vi "GUI Module.vi"(8 "Error In":errorcluster, 10 "GUI Types":T2=enum."Vibratome GUI", 11 "GUI Actions":T1) -> (0 "Error Out":errorcluster)   [LabVIEW 2014]
uses:
  Controls/GUI Types.ctl
  Controls/GUI Module Actions.ctl
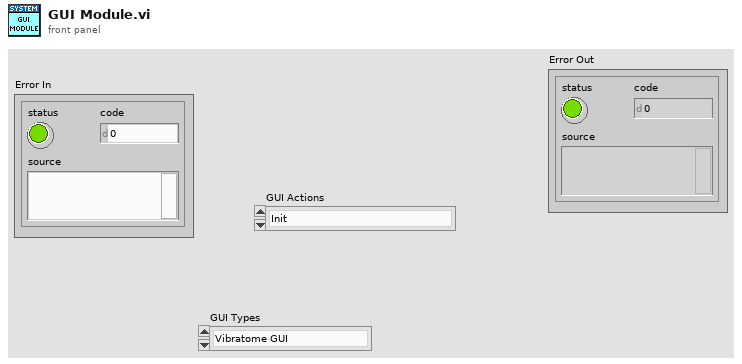
[diagram p1: front panel]
types:
  T1 = typedef "GUI Module Actions.ctl" = enum16{"Init", "Open Front Panel", "Hide All Front Panels", "Close Front Panel", "Uninit"}
  T2 = typedef "GUI Types.ctl" = enum16{"Mosaic GUI", "Vibratome GUI"}
  T3 = enum32{"Invalid", "Standard", "Closed", "Hidden", "Minimized", "Maximized"}
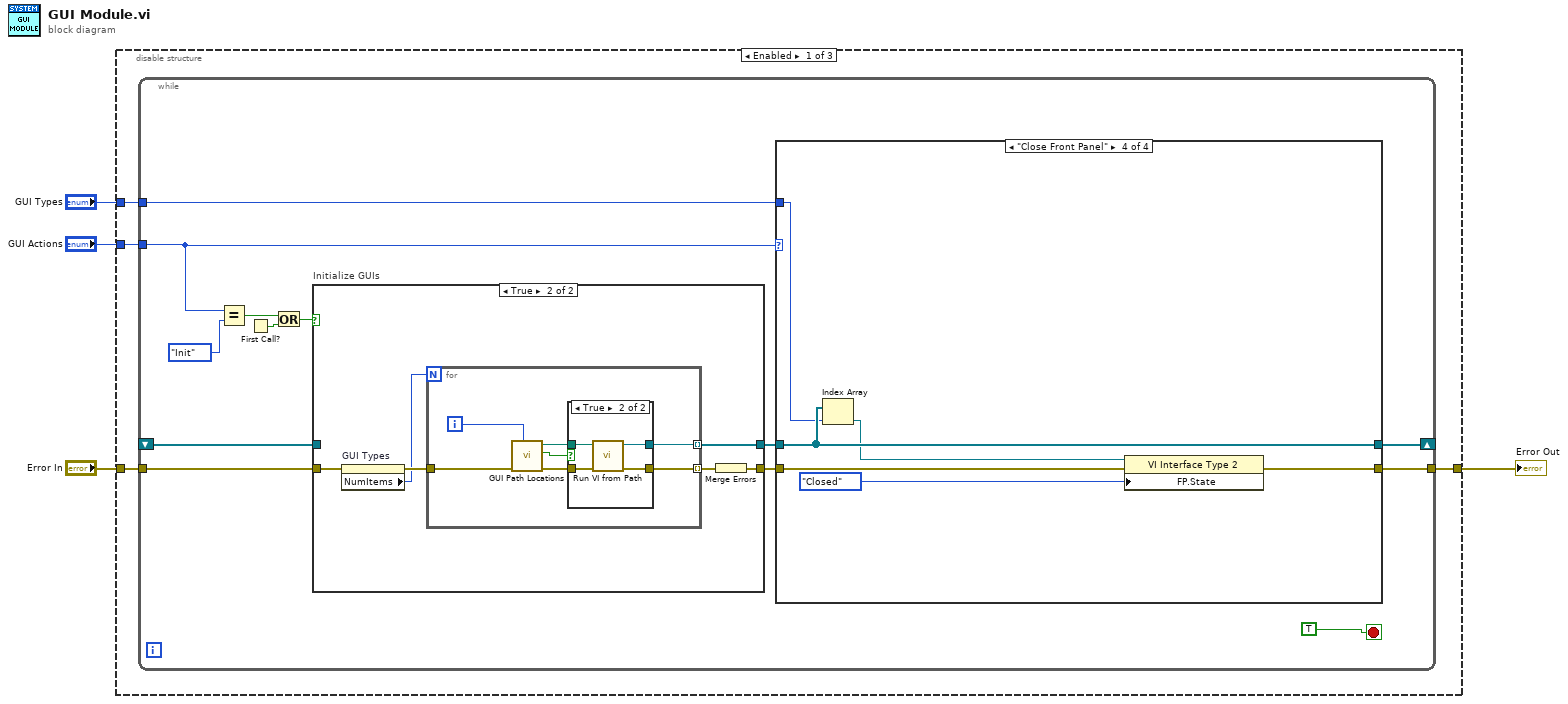
[diagram p0: block diagram]
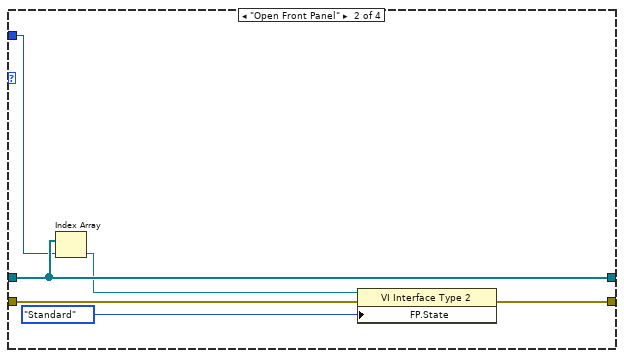
[diagram p3: hidden frame]
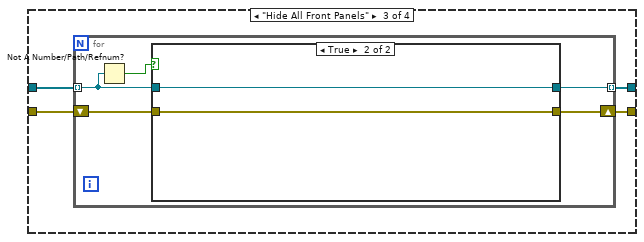
[diagram p4: hidden frame]
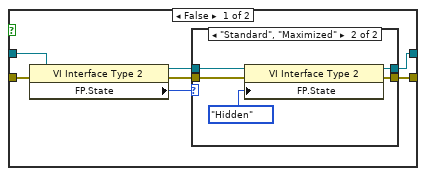
[diagram p5: hidden frame]
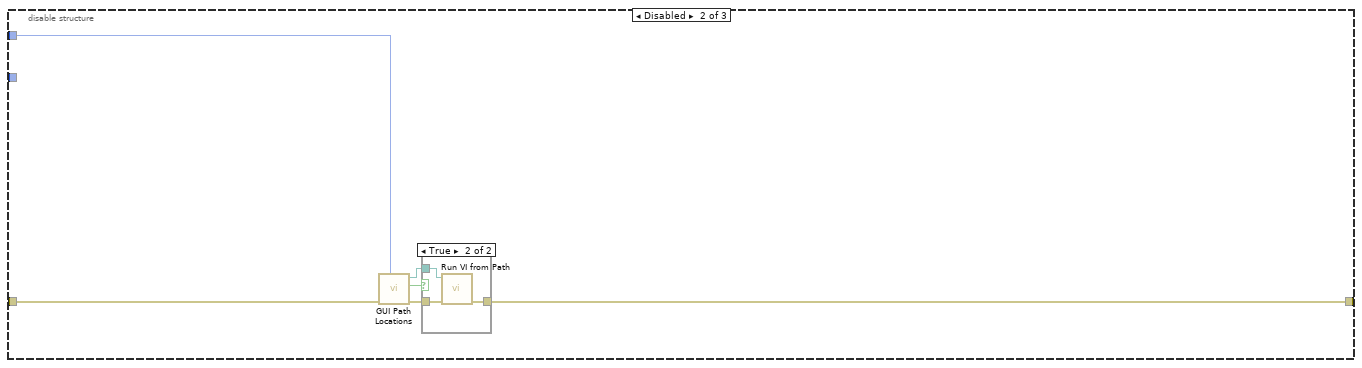
[diagram p9: hidden frame]
diagram:
  n1 = disable-structure shown="Enabled" {
    disable-tunnel: "Error In" -> [w6 w83 w91]
    disable-tunnel: [w5 w82 w91] -> w3
    disable-tunnel: "GUI Types" -> [w8 w81 _]
    disable-tunnel: "GUI Actions" -> [w7 _ _]
    frame Enabled {
      n2 = while {
        tunnel: w7 -> [w12]
        tunnel: w8 -> [w9]
        tunnel: w6 -> [w16]
        tunnel: [w14] -> w5
        shift-right: [w11] -> _
        shift-left: _ -> [w15]
        stop <- TRUE stop-if-true
        n3 = Equal?(x=w12, y=GUI_Module_Actions."Init" ("x")) -> (x = y?=w18:bool)
        n4 = First Call?() -> (First Call?: T/F=w20:bool)
        n5 = Or(x=w18, y=w20) -> (x .or. y?=w19:bool)
        n6 = case "Initialize GUIs" shown="True" w19 {
          tunnel: [w62 w67] -> w13
          tunnel: w16 -> [w62 w66]
          tunnel: [w61 w63] -> w10
          tunnel: w15 -> [w61 _]
          frame False {
          }
          frame True {
            n7 = property on="GUI Types" class="Enum (strict)"(error in=w66) -> (error out=w65:errorcluster, "NumItems"=w64:u32)  [unwired: 1 in, 1 out]
            n8 = for {
              N: w64 -> [_]
              tunnel: [w73] -> w68 mode=indexing
              tunnel: w65 -> [w75]
              tunnel: [w70] -> w63 mode=indexing
              i -> [w69]
              n9 = call "GUI Path Locations.vi"("Enum"=w69, "Error In"=w75) -> ("Error Out"=w74:errorcluster, "file or folder exists?"=w72:bool, "GUI Path"=w71:path)  [unwired: 7 in]
              n10 = case shown="True" w72 {
                tunnel: w74 -> [w76 w80]
                tunnel: [w76 w79] -> w73
                tunnel: w71 -> [_ w78]
                tunnel: [_ w77] -> w70
                frame False {
                }
                frame True {
                  n11 = call "Run VI from Path.vi"("error in (no error)"=w80, "vi path"=w78) -> ("error out"=w79:errorcluster, "type specifier VI Refnum (for type only)"=w77:refnum<vi>)  [unwired: 8 in]
                }
              }
            }
            n12 = Merge Errors(w68) -> (w67:errorcluster)
          }
        }
        n13 = case shown="\"Close Front Panel\"" w12 {
          tunnel: [w22 w28 w32 w59] -> w14
          tunnel: w13 -> [w22 w29 w33 w60]
          tunnel: [w23 w27 w30 w58] -> w11
          tunnel: w10 -> [w23 w27 w31 w58]
          tunnel: w9 -> [_ w26 _ w57]
          frame "Init", Default {
          }
          frame "Open Front Panel" {
            n14 = Index Array(array=w27, index=w26) -> (element=w25:refnum<vi>)
            n15 = property class="VI Interface Type 2"(reference=w25, error in=w29, "FP.State"=T3."Standard" ("Front Panel Window:State")) -> (error out=w28:errorcluster)  [unwired: 1 out]
          }
          frame "Hide All Front Panels" {
            n16 = for {
              shift-right: [w37] -> w32
              shift-left: w33 -> [w38]
              tunnel: w31 -> [w35] mode=indexing
              tunnel: [w36] -> w30 mode=indexing
              n17 = Not A Number/Path/Refnum?(number/path/refnum=w35) -> (NaN/Path/Refnum?=w34:bool)
              n18 = case shown="True" w34 {
                tunnel: w38 -> [w45 w54]
                tunnel: [w44 w54] -> w37
                tunnel: [w43 w53] -> w36
                tunnel: w35 -> [w41 w53]
                frame False {
                  n19 = property class="VI Interface Type 2"(reference=w41, error in=w45) -> (reference out=w40:refnum<vi>, error out=w42:errorcluster, "FP.State"=w39:T3)
                  n20 = case shown="\"Standard\", \"Maximized\"" w39 {
                    tunnel: [w47 w52] -> w44
                    tunnel: [w46 w50] -> w43
                    tunnel: w42 -> [w47 w49]
                    tunnel: w40 -> [w46 w48]
                    frame "Invalid", Default {
                    }
                    frame "Standard", "Maximized" {
                      n21 = property class="VI Interface Type 2"(reference=w48, error in=w49, "FP.State"=T3."Hidden" ("Front Panel Window:State")) -> (reference out=w50:refnum<vi>, error out=w52:errorcluster)
                    }
                  }
                }
                frame True {
                }
              }
            }
          }
          frame "Close Front Panel" {
            n22 = Index Array(array=w58, index=w57) -> (element=w56:refnum<vi>)
            n23 = property class="VI Interface Type 2"(reference=w56, error in=w60, "FP.State"=T3."Closed" ("Front Panel Window:State")) -> (error out=w59:errorcluster)  [unwired: 1 out]
          }
        }
      }
    }
    frame Disabled {
      n24 = call "GUI Path Locations.vi"("Enum"=w81, "Error In"=w83) -> ("Error Out"=w86:errorcluster, "file or folder exists?"=w84:bool, "GUI Path"=w85:path)  [unwired: 7 in]
      n25 = case shown="True" w84 {
        tunnel: w85 -> [_ w89]
        tunnel: w86 -> [w87 w90]
        tunnel: [w87 w88] -> w82
        frame False {
        }
        frame True {
          n26 = call "Run VI from Path.vi"("error in (no error)"=w90, "vi path"=w89) -> ("error out"=w88:errorcluster)  [unwired: 8 in, 1 out]
        }
      }
    }
    frame Disabled {
    }
  }
  "Error Out" <- w3
